vi "PlotDataTypesOut.vi"() -> (1 "point 2":cluster{"x":i16, "y":i16}={"x"=200, "y"=120}, 4 "rect":T4={"left"=45, "top"=45, "right"=200, "bottom"=200}, 5 "point":cluster{"x":i16, "y":i16}={"x"=12, "y"=34}, 6 "alignment":T1, 7 "desired font":T3(ring), 8 "user-specified font":T2={"Font Name:"="Times New Roman", "Size"=36, "Strikeout?"=FALSE, "Italic?"=FALSE, "Underline?"=FALSE, "Outline?"=TRUE, "Shadow?"=TRUE, "Bold?"=TRUE})   [LabVIEW 2010]
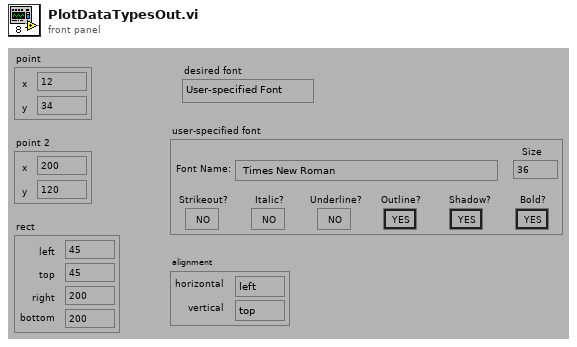
[diagram p1: front panel]
types:
  T1 = cluster{"horizontal":enum16{"left", "center", "right"}, "vertical":enum16{"top", "center", "bottom"}}
  T2 = cluster{"Font Name:":string, "Size":i16, "Strikeout?":bool, "Italic?":bool, "Underline?":bool, "Outline?":bool, "Shadow?":bool, "Bold?":bool}
  T3 = enum16{"User-specified Font", "Application Font", "System Font", "Dialog Font"}
  T4 = cluster{"left":i16, "top":i16, "right":i16, "bottom":i16}
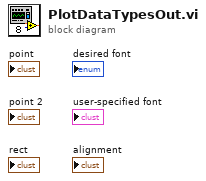
[diagram p0: block diagram]
diagram:
